vi "Magazine_Set.vi"   [LabVIEW 2019]
uses:
  Globals/Magazine_Globals.vi
types:
  T1 = enum16{"No-Op", "Loading", "Fire", "Unjam", "Manual"}
  T2 = typedef "Magazine_Cluster.ctl" = cluster{"Control_States":enum16{"No-Op", "Loading", "Fire", "Unjam", "Manual"}, "Fire":bool, "Magazine_Throttle":dbl}
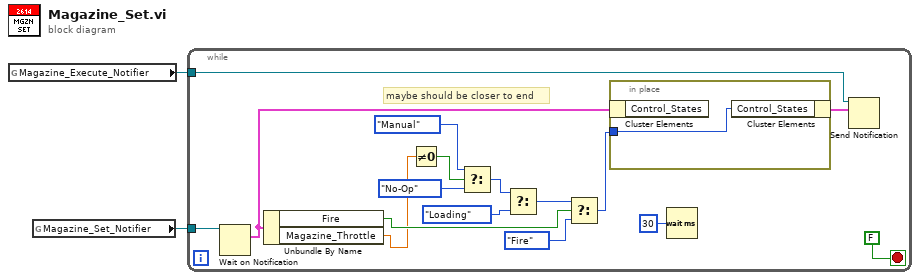
[diagram p0: block diagram]
diagram:
  n1 = global read "Magazine_Globals.vi" "Magazine_Execute_Notifier"() -> (w1:refnum<notifier>)
  n2 = global read "Magazine_Globals.vi" "Magazine_Set_Notifier"() -> (w2:refnum<notifier>)
  n3 = while {
    tunnel: w2 -> [w17]
    tunnel: w1 -> [w16]
    stop <- FALSE stop-if-true
    # "maybe should be closer to end"
    n4 = Wait on Notification(notifier=w17) -> (notification=w14:T2)  [unwired: 3 in, 3 out]
    n5 = Unbundle By Name(w14) -> ("Fire"=w9:bool, "Magazine_Throttle"=w3:dbl)
    n6 = Not Equal To 0?(x=w3) -> (x != 0?=w11:bool)
    n7 = Select(t=T1."Manual" ("Control_States"), s=w11, f=T1."No-Op" ("Control_States")) -> (s? t:f=w12:T1)
    n8 = Select(t=w12, f=T1."Loading" ("Control_States")) -> (s? t:f=w13:T1)  [unwired: 1 in]
    n9 = Select(t=w13, s=w9, f=T1."Fire" ("Control_States")) -> (s? t:f=w5:T1)
    n10 = in-place {
      in-place-border: w5 -> [w19]
      n11 = in-place-cluster #1(w14) -> ()  [unwired: 1 out]
      n12 = in-place-cluster #1("Control_States"=w19) -> (w15:T2)
    }
    n13 = Wait (ms)(milliseconds to wait=u32 30) -> ()  [unwired: 1 out]
    n14 = Send Notification(notification=w15, notifier=w16) -> ()  [unwired: 1 in, 2 out]
  }
